vi "Handle getAll.vi"(8 "error in (no error)":errorcluster, 11 "Instrument.SR7270 in":refnum<class "Instrument.SR7270.lvclass">) -> (0 "error out":errorcluster, 2 "getAll":variant, 3 "Instrument.SR7270 out":refnum<class "Instrument.SR7270.lvclass">)   [LabVIEW 2019, in "Instrument.SR7270.lvclass"]
uses:
  Instrument.SR7270.lvclass
  Instrument.SR7270.lvclass/Instrument.SR7270.ctl
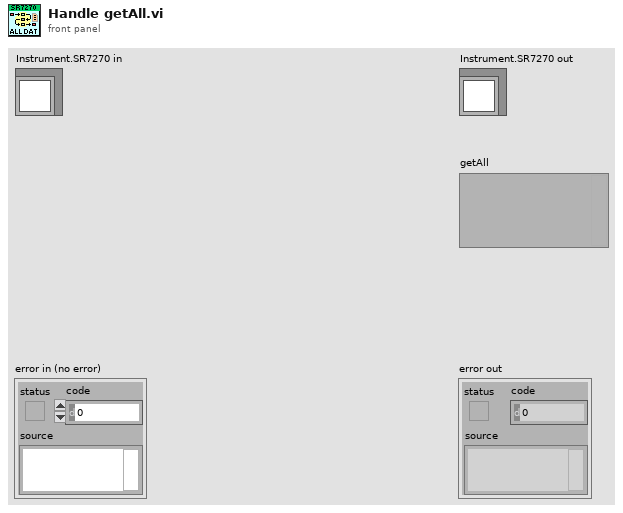
[diagram p1: front panel]
types:
  T1 = typedef "Instrument.SR7270.lvclass/getAll.ctl" = cluster{"X (V or A)":dbl, "Y (V or A)":dbl, "Mag (V or A)":dbl, "Phase (°)":dbl, "Oscillator Amplitude (V)":dbl, "Oscillator frequency (Hz)":dbl, "REF time constant (s)":dbl, "REF harmonic":u16, "REF phase (°)":dbl, "REF frequency (Hz)":dbl, "AC Gain":string, "Current Mode":string, "AC-DC Coupling":string, "FET":string, "Float":string, "Line Filter":string, "Voltage Mode":string, "Sensitivity (V or A)":dbl}
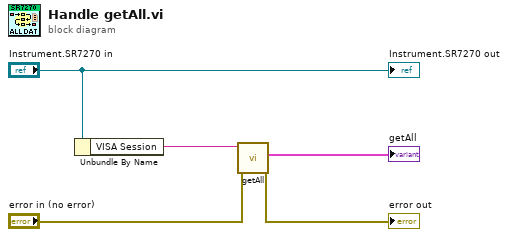
[diagram p0: block diagram]
diagram:
  n1 = Unbundle By Name("Instrument.SR7270 in") -> ("VISA Session"=w5:string)
  n2 = call "getAll.vi"("error in (no error)"="error in (no error)", "VISA Session"=w5) -> ("error out"=→"error out":errorcluster, "SR7270 getAll"=→"getAll":T1)  [unwired: 7 in, 1 out]
  "Instrument.SR7270 out" <- "Instrument.SR7270 in"
